vi "Read Annotations in timeframe.vi"(8 "error in (no error)":errorcluster, 10 "End Time":timestamp, 11 "Start Time":timestamp) -> (0 "error out":errorcluster)   [LabVIEW 2011]
doc: "This VI reads all event files in the project folder. It loads all annotations that has occurred during the buffer length."
uses:
  emi Lib/System 01/0 - General/S&E reporting/Private/_emi_ S&E Message.ctl
  emi Lib/System 01/0 - General/S&E reporting/Private/_emi_ S&E Message type.ctl
  Actin Annotatino Holder.ctl
  Annotation Message.ctl
  emi cndiates/E&S/reate/S&E Anotationtype.ctl
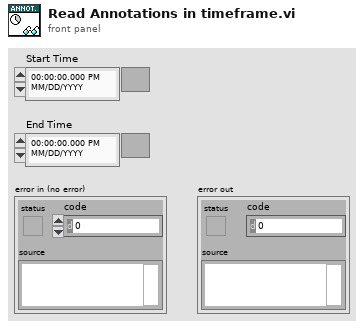
[diagram p1: front panel]
types:
  T1 = typedef "Actin Annotatino Holder.ctl" = enum16{"GET Single", "GET All", "GET Time Period", "GET Index", "Get Size", "Add Single", "Replace Single", "Delete Single", "SET All"}
  T2 = typedef "_emi_ S&E Message.ctl" = cluster{"Type":T3, "Originate time":dbl, "System":u8, "Loop":u16, "Sub ID":u16, "Elevated priority":bool, "E&S Message content":variant}
  T3 = typedef "_emi_ S&E Message type.ctl" = enum16{"Error/Warning", "Note", "Debug", "Event", "Alarm Analog", "Alarm Digital", "Annotation"}
  T4 = typedef "Project infor with project path.ctl" = cluster{"Project path":path, "data":T5, "Comment":string}
  T5 = typedef "Project in icluster.ctl" = cluster{"Job and Site":T6, "Tool":T8, "Run Information":T9}
  T6 = typedef "Job and site cluster.ctl" = cluster{"Project Number":string, "Client Company":string, "Country":T7, "Field":string, "Rig":string, "Well":string}
  T7 = typedef "List of all contrys(combo box).ctl" = string
  T8 = typedef "Tool registration ID.ctl" = cluster{"Tractor type":string, "Tool":string, "Serial #":string}
  T9 = typedef "Run Information.ctl" = cluster{"Active Run":bool, "String Check Rec":bool, "Run Number":i32, "Time of File Start":string}
  T10 = typedef "Annotation Message.ctl" = cluster{"Annotation":string, "User":string, "time":timestamp}
  T11 = typedef "S&E Anotationtype.ctl" = cluster{"User":string, "Annotation":string}
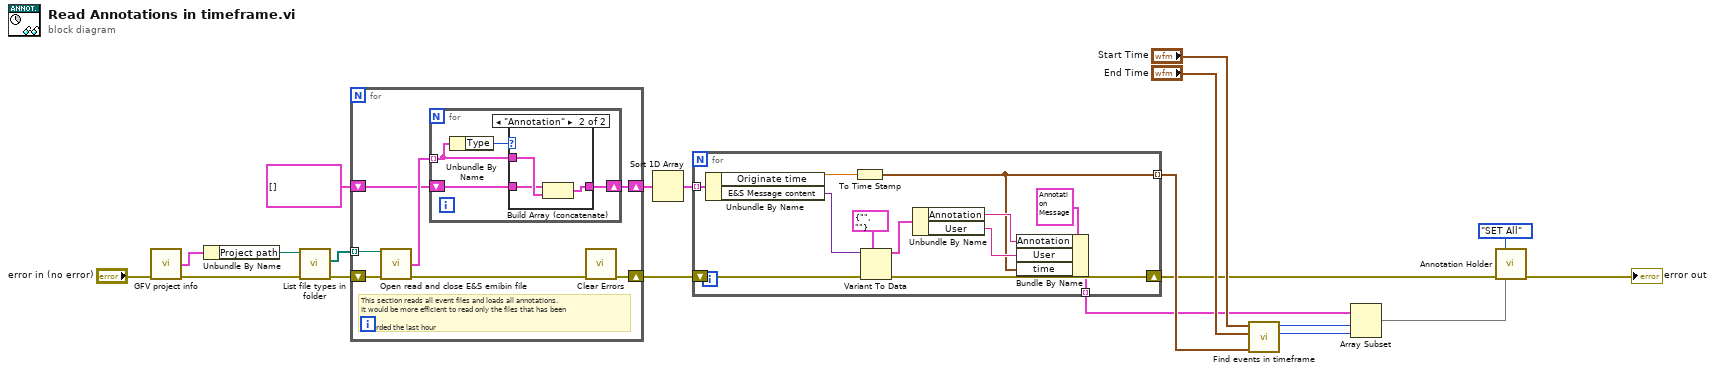
[diagram p0: block diagram]
diagram:
  n1 = call "GFV project info.vi"("error in (no error)"="error in (no error)") -> ("Project info out"=w2:T4, "error out"=w3:errorcluster)  [unwired: 13 in]
  n2 = Unbundle By Name(w2) -> ("Project path"=w1:path)
  n3 = call "List file types in folder.vi"("error in (no error)"=w3, "Project folder"=w1) -> ("error out"=w14:errorcluster, "Binary STAT files"=w13:path[])  [unwired: 7 in, 1 out]
  n4 = for {
    tunnel: w13 -> [w27] mode=indexing
    shift-right: [w25] -> w16
    shift-left: T2[] [] -> [w24]
    shift-right: [w21] -> w10
    shift-left: w14 -> [w23]
    # "This section reads all event files and loads all annotations.\nIt would be more efficient to read only the files that has been\n\nrecorded the last hour"
    n5 = call "Open read and close E&S emibin file.vi"("file path"=w27, "error in"=w23) -> ("E&S records"=w26:T2[], "error out"=w22:errorcluster)  [unwired: 11 in, 1 out]
    n6 = for {
      tunnel: w26 -> [w30] mode=indexing
      shift-right: [w29] -> w25
      shift-left: w24 -> [w28]
      n7 = Unbundle By Name(w30) -> ("Type"=w31:T3)
      n8 = case shown="\"Annotation\"" w31 {
        tunnel: w30 -> [_ w35]
        tunnel: [w32 w34] -> w29
        tunnel: w28 -> [w32 w33]
        frame "Error/Warning", Default {
        }
        frame "Annotation" {
          n9 = Build Array (concatenate)(w33, w35) -> (w34:T2[])
        }
      }
    }
    n10 = call <vilib>:"Clear Errors.vi"("error in (no error)"=w22) -> ("error out"=w21:errorcluster)  [unwired: 6 in]
  }
  n11 = Sort 1D Array(array=w16) -> (sorted array=w17:T2[])
  n12 = for {
    tunnel: w17 -> [w47] mode=indexing
    tunnel: [w37] -> w18 mode=indexing
    shift-right: [w43] -> w6
    shift-left: w10 -> [w42]
    tunnel: [w36] -> w8 mode=indexing
    n13 = Unbundle By Name(w47) -> ("Originate time"=w46:dbl, "E&S Message content"=w44:variant)
    n14 = To Time Stamp(1:w46) -> (0:w37:timestamp)
    n15 = Variant To Data(error in=w42, type=T11 {"User"="", "Annotation"=""} ("S&E Alarm"), Variant=w44) -> (data=w40:T11, error out=w43:errorcluster)
    n16 = Unbundle By Name(w40) -> ("Annotation"=w39:string, "User"=w38:string)
    n17 = Bundle By Name(cluster=T10 {"Annotation"="", "User"="", "time"=timestamp(0 s since 1904-01-01)} ("Annotation out"), "Annotation"=w39, "User"=w38, "time"=w37) -> (w36:T10)
  }
  n18 = call "Find events in timeframe.vi"("Data Array"=w18, "End time"="End Time", "Start time"="Start Time") -> ("length out"=w11:i32, "index out"=w12:i32)  [unwired: 6 in, 1 out]
  n19 = Array Subset(array=w8, index=w12, length=w11) -> (w7:T10[])
  n20 = call "Annotation Holder.vi"("Action"=Actin_Annotatino_Holder."SET All", "error in (no error)"=w6, "Array of annotations in"=w7) -> ("error out"=→"error out":errorcluster)  [unwired: 8 in, 4 out]
